vi "FPGA_MAIN_lock-in-1.vi"() -> ()   [LabVIEW 2013]
uses:
  <vilib>/rvi/FIFO/Fifo_Resource/nirvififoEmulationClearFpgaImpl.vi
  <vilib>/rvi/DataTransferAndStorage/Container/Common/niFpgaContainerGetUniqueNameForEmu.vi
  <vilib>/rvi/eio/common/nirviEmuTemplateMethod_errors.vi
  <vilib>/rvi/Emulation/niFpgaSctlEmulationGetInTimedLoop.vi
  <vilib>/rvi/Emulation/niFpgaEmulationReportErrorSimple.vi
  <vilib>/rvi/Emulation/niFpgaGetClockAttributes.vi
  <vilib>/rvi/Emulation/niFpgaCriticalErrorInLSC.vi
  <vilib>/rvi/Memory/Memory_Emulation/nirvimemoryEmulation.vi
  <vilib>/rvi/Memory/Memory_Emulation/nirvimemoryFastEmulation.vi
  <vilib>/rvi/Memory/Memory_Emulation/niFpgaMemoryEmulationCacheClearOnFirstRun.vi
  <vilib>/rvi/Memory/Memory_Emulation/nirvimemoryEmulationManagerCache_MakeExclusive.vi
  <vilib>/rvi/Memory/Memory_Emulation/niFpgaMemoryEmulationValidateCache.vi
  <vilib>/rvi/Memory/Memory_Emulation/nirvimemoryEmulationManagerCache_ReleaseExclusive.vi
  <vilib>/rvi/Memory/Memory_Emulation/nirvimemoryEmulationManagerCache_InsertValue.vi
  <vilib>/Utility/error.llb/Clear Errors.vi
  <vilib>/rvi/Memory/Memory_Emulation/nirvimemoryEmulationManagerCache_GetValue.vi
  <vilib>/rvi/Emulation/niFpgaProcessEmulError.vi
  <vilib>/rvi/FIFO/Fifo_Resource/nirvififoEmulationReadFpgaImpl.vi
  <vilib>/rvi/FIFO/Fifo_Resource/nirvififoEmulationWriteFpgaImpl.vi
  <vilib>/rvi/DataTransferAndStorage/Container/XNode/niFpgaContainer.xnode
  <vilib>/rvi/FIFO/Fifo_Resource/nirvififoEmulationClear.vi
  <vilib>/eio/EIONode/EIONode.xnode
  <vilib>/rvi/FIFO/Fifo_Resource/nirvififoEmulationRead.vi
  <vilib>/rvi/FIFO/Fifo_Resource/nirvififoEmulationWrite.vi
panel:
  in  "DAC to retrieve":u16
  in  "got DAC value":bool
  out "DAC data":u32
  out "get DAC value":bool
  out "move bus ready":bool=TRUE
  out "sending order":bool
  out "subsystem":u8
  in  "order in":u64
  in  "order Xmitted":bool
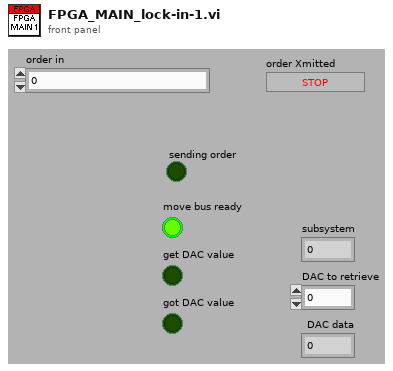
[diagram p1: front panel]
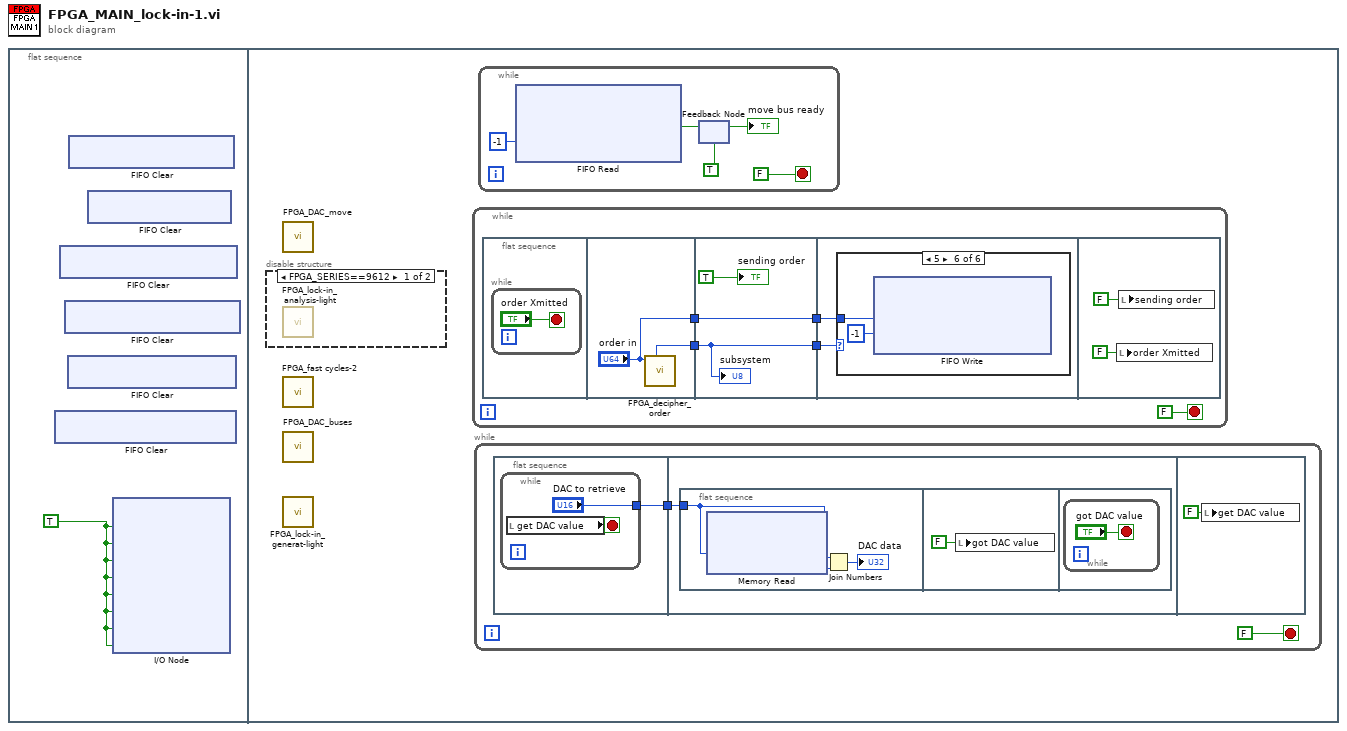
[diagram p0: block diagram]
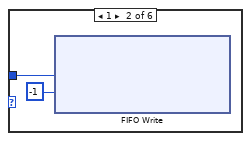
[diagram p4: hidden frame]
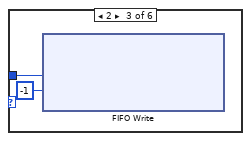
[diagram p5: hidden frame]
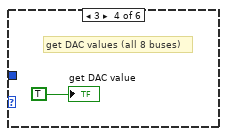
[diagram p6: hidden frame]
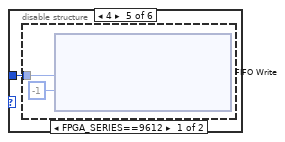
[diagram p7: hidden frame]
diagram:
  n1 = flat-sequence {
    frame #0 {
      w1 = TRUE ("Port0/DIOCTL")
      n2 = xnode ("FIFO Clear")() -> ()  [unwired: 1 in, 1 out]
      n3 = xnode ("FIFO Clear")() -> ()  [unwired: 1 in, 1 out]
      n4 = xnode ("FIFO Clear")() -> ()  [unwired: 1 in, 1 out]
      n5 = xnode ("FIFO Clear")() -> ()  [unwired: 1 in, 1 out]
      n6 = xnode ("FIFO Clear")() -> ()  [unwired: 1 in, 1 out]
      n7 = xnode ("FIFO Clear")() -> ()  [unwired: 1 in, 1 out]
      n8 = xnode "I/O Node"("Port0/DIOCTL"=w1, "Port1/DIOCTL"=w1, "Port2/DIOCTL"=w1, "Port3/DIOCTL"=w1, "Port4/DIOCTL"=w1, "Port5/DIOCTL"=w1, "Port6/DIOCTL"=w1, "Port7/DIOCTL"=w1) -> ()  [unwired: 8 in, 8 out]
    }
    frame #1 {
      n9 = disable-structure shown="FPGA_SERIES==9612" {
        frame condition #0 {
          n10 = call "FPGA_lock-in_analysis-light.vi"() -> ()  [unwired: 1 out]
        }
        frame condition #1 (active) {
        }
      }
      n11 = call "FPGA_DAC_move.vi"() -> ()  [unwired: 12 out]
      n12 = call "FPGA_fast cycles-2.vi"() -> ()  [unwired: 1 out]
      n13 = call "FPGA_DAC_buses.vi"() -> ()  [unwired: 12 out]
      n14 = call "FPGA_lock-in_generat-light.vi"() -> ()  [unwired: 1 out]
      n15 = while {
        stop <- FALSE stop-if-true
        n16 = flat-sequence {
          tunnel: [w26] -> w21
          tunnel: ["order in"] -> w19
          tunnel: [w29] -> w22
          tunnel: w21 -> [w29]
          tunnel: [w27] -> w20
          tunnel: w19 -> [w27]
          tunnel: w22 -> [w31]
          tunnel: w20 -> [w30]
          frame #0 {
            n17 = while {
              stop <- "order Xmitted" stop-if-true
            }
          }
          frame #1 {
            n18 = call "FPGA_decipher_order.vi"("order in"="order in") -> ("subsystem"=w26:u8)  [unwired: 10 out]
          }
          frame #2 {
            "sending order" <- TRUE ("Boolean")
            "subsystem" <- w29
          }
          frame #3 {
            n19 = case shown="5" w31 {
              tunnel: w30 -> [_ w33 w35 _ w37 w41]
              frame 0, Default {
              }
              frame 1 {
                n20 = xnode ("FIFO Write")("Element"=w33, "Timeout"=-1) -> ()  [unwired: 1 in, 2 out]
              }
              frame 2 {
                n21 = xnode ("FIFO Write")("Element"=w35, "Timeout"=-1) -> ()  [unwired: 1 in, 2 out]
              }
              frame 3 {
                # "get DAC values (all 8 buses)"
                "get DAC value" <- TRUE ("get DAC values")
              }
              frame 4 {
                n22 = disable-structure shown="FPGA_SERIES==9612" {
                  disable-tunnel: w37 -> [w39 _]
                  frame condition #0 {
                    n23 = xnode ("FIFO Write")("Element"=w39, "Timeout"=-1) -> ()  [unwired: 1 in, 2 out]
                  }
                  frame condition #1 (active) {
                  }
                }
              }
              frame 5 {
                n24 = xnode ("FIFO Write")("Element"=w41, "Timeout"=-1) -> ()  [unwired: 1 in, 2 out]
              }
            }
          }
          frame #4 {
            n25 = local write "order Xmitted"(FALSE ("order Xmitted")) -> ()
            n26 = local write "sending order"(FALSE ("sending order")) -> ()
          }
        }
      }
      n27 = while {
        stop <- FALSE stop-if-true
        n28 = flat-sequence {
          tunnel: [w4] -> w2
          tunnel: w2 -> [w7]
          frame #0 {
            n29 = while {
              tunnel: ["DAC to retrieve"] -> w4
              stop <- w6 stop-if-true
              n30 = local read "get DAC value"() -> (w6:bool)
            }
          }
          frame #1 {
            n31 = flat-sequence {
              tunnel: w7 -> [w8]
              frame #0 {
                n32 = xnode ("Memory Read")("Address"=w8) -> ("Data"=w10:u16)  [unwired: 1 in, 1 out]
                n33 = Join Numbers(hi=w8, lo=w10) -> ((hi.lo)=→"DAC data":u32)
              }
              frame #1 {
                n34 = local write "got DAC value"(FALSE ("got DAC value")) -> ()
              }
              frame #2 {
                n35 = while {
                  stop <- "got DAC value" stop-if-true
                }
              }
            }
          }
          frame #2 {
            n36 = local write "get DAC value"(FALSE ("get DAC values")) -> ()
          }
        }
      }
      n37 = while {
        stop <- FALSE stop-if-true
        n38 = xnode ("FIFO Read")("Timeout"=-1) -> ("Element"=w17:bool)  [unwired: 1 in, 2 out]
        n39 = feedback-in #1(w17) -> ()
        n40 = feedback #1(TRUE ("Element")) -> (→"move bus ready":bool)
      }
    }
  }
